vi "To Variant.vi"(0 "Obj in":refnum<class "TCPController.lvclass">, 11 "error in (no error)":errorcluster) -> (4 "Obj out":refnum<class "TCPController.lvclass">, 8 "Array":variant[](array[variant]), 15 "error out":errorcluster)   [LabVIEW 2020, in "TCPController.lvclass"]
uses:
  TCPController.lvclass
  TCPController.lvclass/TCPController.ctl
  Base Class/TTLController.lvclass
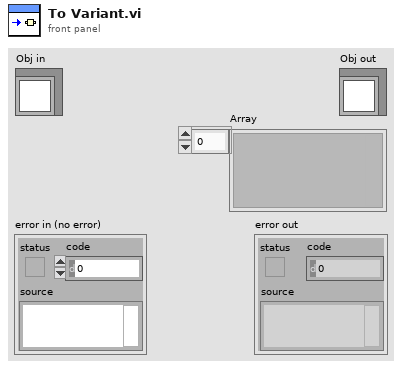
[diagram p1: front panel]
types:
  T1 = typedef "TCPController.lvclass/Serialized.ctl" = cluster{"Numeric":dbl}
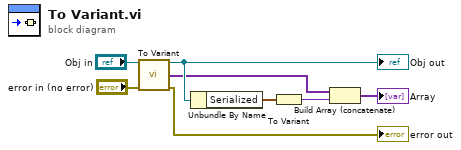
[diagram p0: block diagram]
diagram:
  n1 = call-parent "To Variant.vi"("TTLController in"="Obj in", "error in (no error)"="error in (no error)") -> ("TTLController out"=w3:refnum<class "TCPController.lvclass">, "Array"=w2:variant[], "error out"=→"error out":errorcluster)  [unwired: 11 in]
  "Obj out" <- w3
  n2 = Unbundle By Name(w3) -> ("Serialized"=w4:T1)
  n3 = To Variant(anything=w4) -> (Variant=w5:variant)
  n4 = Build Array (concatenate)(w2, w5) -> (→"Array":variant[])
